vi "BRig_RT__Case_Exp__storeData__endExp.vi"(0 "input_dataBlock":u16[][](array[numeric]), 1 "input_dataCurrent":u16[](array[numeric]), 2 "input_dataLick":u16[][](array[numeric]), 5 "input_dataTrial":u16[][](array[numeric]), 7 "input_dataExp":u16[](array[numeric]), 9 "input_dataLC":u16[](array[numeric]), 11 "input_dataMTrig":u16[](array[numeric]), 12 "input_dataAnalog":u16[][](array[numeric]), 13 "input_dataAnalog_length":i32) -> ()   [LabVIEW 2014]
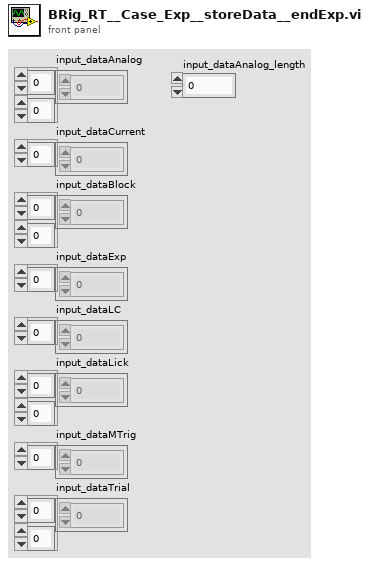
[diagram p1: front panel]
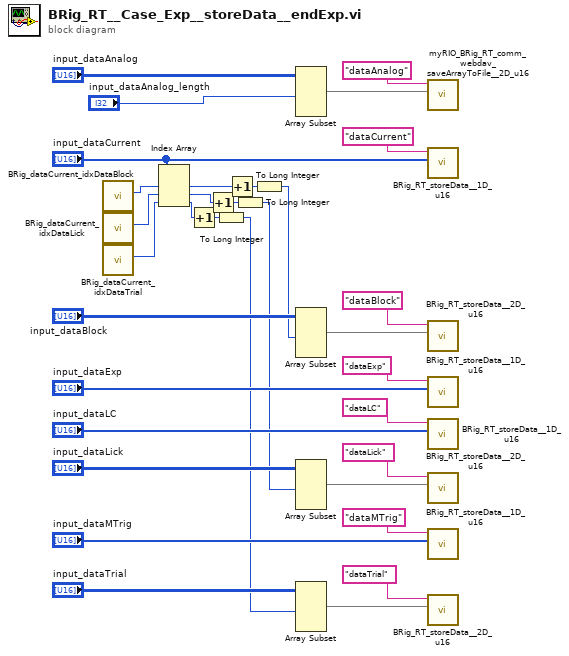
[diagram p0: block diagram]
diagram:
  n1 = call "BRig_dataCurrent_idxDataBlock.vi"() -> ("output_idxDataBlock"=w31:i32)  [unwired: 11 in]
  n2 = call "BRig_dataCurrent_idxDataLick.vi"() -> ("output_idxDataLick"=w30:i32)  [unwired: 11 in]
  n3 = call "BRig_dataCurrent_idxDataTrial.vi"() -> ("output_idxDataTrial"=w29:i32)  [unwired: 11 in]
  n4 = Index Array(array="input_dataCurrent", index #1=w31, index #2=w30, index #3=w29) -> (element #1=w25:u16, element #2=w22:u16, element #3=w19:u16)
  n5 = Increment(x=w19) -> (x+1=w20:u16)
  n6 = Increment(x=w22) -> (x+1=w21:u16)
  n7 = To Long Integer(number=w20) -> (32bit integer=w5:i32)
  n8 = Increment(x=w25) -> (x+1=w24:u16)
  n9 = To Long Integer(number=w21) -> (32bit integer=w11:i32)
  n10 = To Long Integer(number=w24) -> (32bit integer=w23:i32)
  n11 = Array Subset(array="input_dataAnalog", length (row)="input_dataAnalog_length") -> (w3:u16[][])  [unwired: 3 in]
  n12 = Array Subset(array="input_dataBlock", length (row)=w23) -> (w27:u16[][])  [unwired: 3 in]
  n13 = Array Subset(array="input_dataLick", length (row)=w11) -> (w14:u16[][])  [unwired: 3 in]
  n14 = Array Subset(array="input_dataTrial", length (row)=w5) -> (w8:u16[][])  [unwired: 3 in]
  n15 = call "myRIO_BRig_RT_comm_webdav_saveArrayToFile__2D_u16.vi"("Array"=w3, "input_filename"="dataAnalog") -> ()  [unwired: 10 in]
  n16 = call "BRig_RT_storeData__1D_u16.vi"("Array"="input_dataCurrent", "input_filename"="dataCurrent") -> ()  [unwired: 10 in]
  n17 = call "BRig_RT_storeData__2D_u16.vi"("Array"=w27, "input_filename"="dataBlock") -> ()  [unwired: 10 in]
  n18 = call "BRig_RT_storeData__1D_u16.vi"("Array"="input_dataExp", "input_filename"="dataExp") -> ()  [unwired: 10 in]
  n19 = call "BRig_RT_storeData__1D_u16.vi"("Array"="input_dataLC", "input_filename"="dataLC") -> ()  [unwired: 10 in]
  n20 = call "BRig_RT_storeData__2D_u16.vi"("Array"=w14, "input_filename"="dataLick") -> ()  [unwired: 10 in]
  n21 = call "BRig_RT_storeData__1D_u16.vi"("Array"="input_dataMTrig", "input_filename"="dataMTrig") -> ()  [unwired: 10 in]
  n22 = call "BRig_RT_storeData__2D_u16.vi"("Array"=w8, "input_filename"="dataTrial") -> ()  [unwired: 10 in]
